vi "init.vi"(8 "error in (no error)":errorcluster, 11 "PressureTransducerCompensator in":refnum<class "PressureTransducerCompensator.lvclass">) -> (0 "error out":errorcluster, 3 "PressureTransducerCompensator out":refnum<class "PressureTransducerCompensator.lvclass">)   [LabVIEW 2013, in "PressureTransducerCompensator.lvclass"]
uses:
  PressureTransducerCompensator.lvclass
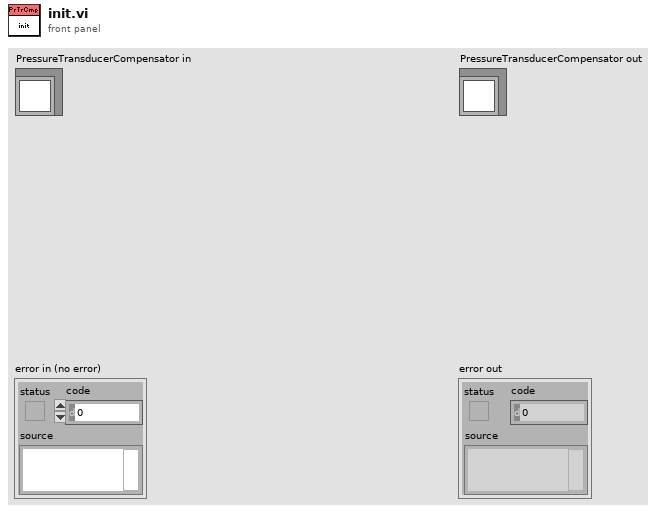
[diagram p1: front panel]
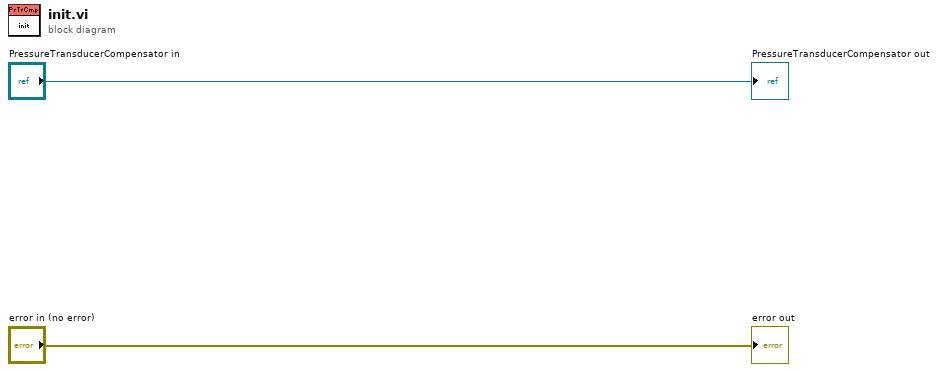
[diagram p0: block diagram]
diagram:
  "error out" <- "error in (no error)"
  "PressureTransducerCompensator out" <- "PressureTransducerCompensator in"
